vi "specu1a 1.0.0 Read Parameters.vi"(3 "error in (no error)":errorcluster, 5 "Device Handle":i32) -> (0 "error out":errorcluster, 1 "Parameters":T1={"Integration time"=10000, "Gain"=enum."Low", "TriggerEdge"=enum."Rising", "Trigger Mode"=enum."Internal", "Reserved"=0}, 2 "Device Handle out":i32)   [LabVIEW 2019]
uses:
  Controls/specu1a 1.0.0 Parameters.ctl
  Controls/specu1a 1.0.0 Trigger Edge.ctl
  Controls/specu1a 1.0.0 Trigger Mode.ctl
  WINDOWS/SYSTEM32/DRIVERS/specu1a.dll
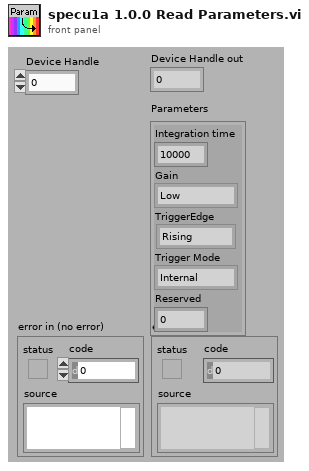
[diagram p1: front panel]
types:
  T1 = typedef "specu1a 1.0.0 Parameters.ctl" = cluster{"Integration time":u32, "Gain":enum16{"Low", "High", "No Function"}, "TriggerEdge":T2, "Trigger Mode":T3, "Reserved":u8}
  T2 = typedef "specu1a 1.0.0 Trigger Edge.ctl" = enum16{"Rising", "Falling", "No Function"}
  T3 = typedef "specu1a 1.0.0 Trigger Mode.ctl" = enum16{"Internal", "Asynchronous", "Synchronous"}
  T4 = cluster{"Integration time":u32, "Gain":u8, "Trigger edge":u8, "Trigger mode":u8, "Reserved":u8}
  T5 = typedef "specu1a 1.0.0 Error codes.ctl" = enum16{"INVALID_HANDLE_VALUE", "USBDEV_SUCCESS", "USBDEV_INVALID_HANDLE", "USBDEV_UNSUCCESS", "USBDEV_INVALID_VALUE", "USBDEV_CHECK_NORMAL", "USBDEV_CHECK_INVALID", "USBDEV_CHECK_REMOVE", "USBDEV_CHECK_OTHER", "USBDEV_RESET_ERROR", "USBDEV_BULKSIZE_ERROR", "USBDEV_BULK_READ_ERROR", "USBDEV_BULK_NOT_UPDATED", "USBDEV_TIME_OVER_ERROR", "USBDEV_TIME_UNDER_ERROR", "USBDEV_TIME_SET_ERROR", "USBDEV_SET_GAIN_ERROR", "USBDEV_GET_TEMP_ERROR", "USBDEV_SET_TRIGGER_ERROR", "USBDEV_RW_EEP_ADDR_ERROR", "USBDEV_RW_EEP_SIZE_ERROR", "USBDEV_RW_EEP_OVER_ERROR", "USBDEV_RW_EEP_ERROR", "UNITID_PRODUCTID_CONFLICT", "UNKNOWN_ERROR"}
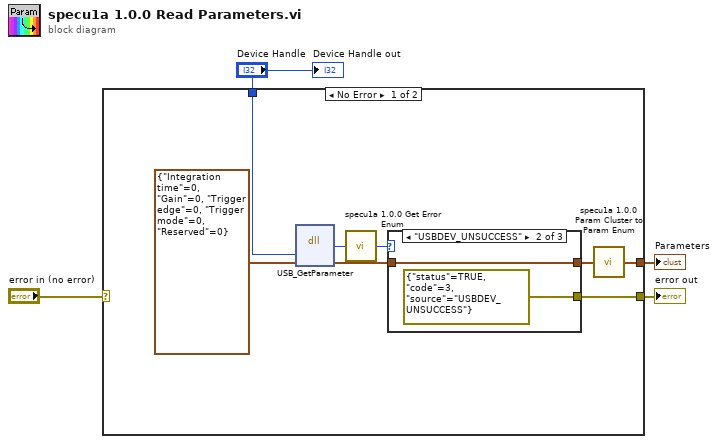
[diagram p0: block diagram]
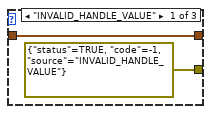
[diagram p2: hidden frame]
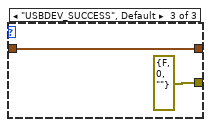
[diagram p3: hidden frame]
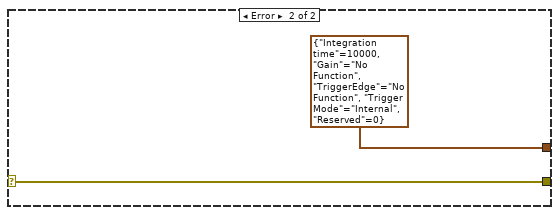
[diagram p4: hidden frame]
diagram:
  n1 = case shown="No Error" "error in (no error)" {
    selector: "error in (no error)" -> [_ w20]
    tunnel: [w11 w20] -> w3
    tunnel: [w5 T1 {"Integration time"=10000, "Gain"=enum."No Function", "TriggerEdge"=enum."No Function", "Trigger Mode"=enum."Internal", "Reserved"=0} ("Parameters")] -> w1
    tunnel: "Device Handle" -> [w10 _]
    frame No Error {
      n2 = dll-call lib="C:/WINDOWS/SYSTEM32/DRIVERS/specu1a.dll" fn="USB_GetParameter" label="1.0.0 GetParameter"("Device Handle"=w10, T4 {"Integration time"=0, "Gain"=0, "Trigger edge"=0, "Trigger mode"=0, "Reserved"=0}) -> (w9:u16, w8:T4)  [unwired: 4 in, 2 out]
      n3 = call "specu1a 1.0.0 Get Error Enum.vi"("Error Code in"=w9) -> ("Specu1a 1.0.0 Error code out"=w12:T5)  [unwired: 4 in]
      n4 = case shown="\"USBDEV_UNSUCCESS\"" w12 {
        tunnel: [w13 w15 w17] -> w6
        tunnel: [errorcluster {"status"=TRUE, "code"=-1, "source"="INVALID_HANDLE_VALUE"} ("error out") errorcluster {"status"=TRUE, "code"=3, "source"="USBDEV_UNSUCCESS"} ("error out") errorcluster {"status"=FALSE, "code"=0, "source"=""} ("error out")] -> w11
        tunnel: w8 -> [w13 w15 w17]
        frame "INVALID_HANDLE_VALUE" {
        }
        frame "USBDEV_UNSUCCESS" {
        }
        frame "USBDEV_SUCCESS", Default {
        }
      }
      n5 = call "specu1a 1.0.0 Param Cluster to Param Enum.vi"("Cluster in"=w6) -> ("Parameters"=w5:T1)
    }
    frame Error {
    }
  }
  "error out" <- w3
  "Parameters" <- w1
  "Device Handle out" <- "Device Handle"
